vi "YAFTAF_UserInterface.vi"(8 "ErrorIn":errorcluster, 11 "ActorClass":refnum<class "YAFTAF.lvclass">) -> ()   [LabVIEW 2021, in "YAFTAF.lvclass"]
uses:
  YAFTAF.lvclass
  YAFTAF.lvclass/YAFTAF.ctl
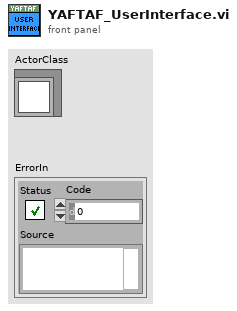
[diagram p1: front panel]
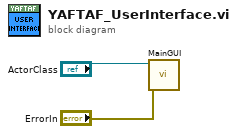
[diagram p0: block diagram]
diagram:
  n1 = call-dynamic "MainGUI.vi"("ErrorIn"="ErrorIn", "ObjectIn"="ActorClass") -> ()  [unwired: 10 in]
